vi "CDMA_Modulation.vi"(7 "ch1_sf_tx":dbl, 8 "error in (no error)":errorcluster caption="错误输入（无错误）", 10 "sf_data":dbl[](array[numeric]), 11 "Path":path) -> (0 "error out":errorcluster caption="错误输出", 1 "data_q":dbl[](array[numeric]), 2 "data_i":dbl[](array[numeric]), 3 "Path Out":path, 4 "output_data":cdb[](array[numeric]))   [LabVIEW 2015]
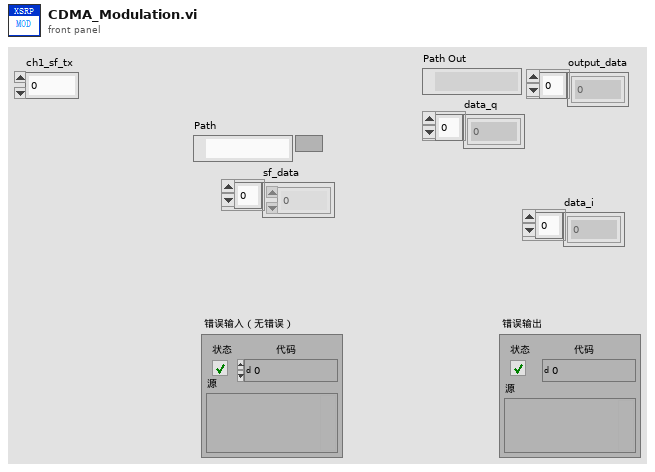
[diagram p1: front panel]
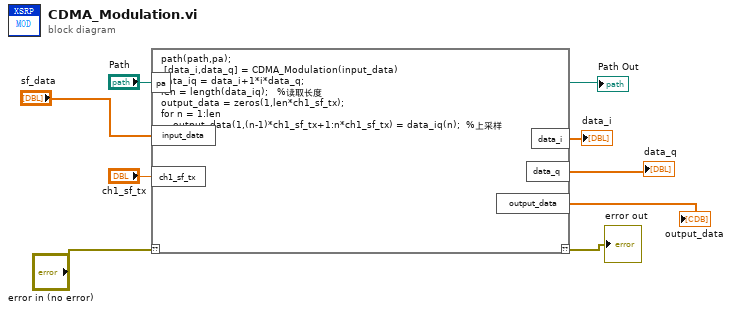
[diagram p0: block diagram]
diagram:
  n1 = script code="path(path,pa);\n [data_i,data_q] = CDMA_Modulation(input_data)\ndata_iq = data_i+1*i*data_q;\nlen = length(data_iq);   %读取长度\noutput_data = zeros(1,len*ch1_sf_tx);\nfor n = 1:len\n    output_data(1,(n-1)*ch1_sf_tx+1:n*ch1_sf_tx) = data_iq(n);  %上采样\nend"("??"="error in (no error)", "pa"="Path", "input_data"="sf_data", "ch1_sf_tx"="ch1_sf_tx") -> ("??"=→"error out":errorcluster, "data_i"=→"data_i":dbl[], "data_q"=→"data_q":dbl[], "output_data"=→"output_data":cdb[])
  "Path Out" <- "Path"
